vi "bcdToInt.vi"(10 "y":u8 format="%x") -> (1 "x .and. y?":u8, 2 "x << y":u8)   [LabVIEW 2019]
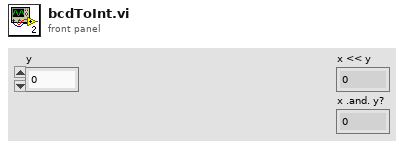
[diagram p1: front panel]
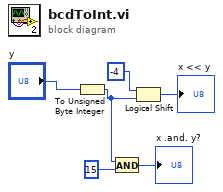
[diagram p0: block diagram]
diagram:
  n1 = To Unsigned Byte Integer(number="y") -> (unsigned 8bit integer=w3:u8)
  n2 = And(x=w3, y=u8 15) -> (x .and. y?=→"x .and. y?":u8)
  n3 = Logical Shift(y=i16 -4, x=w3) -> (x << y=→"x << y":u8)
